vi "录音机实验.vi"() -> ()   [LabVIEW 2011]
uses:
  <vilib>/STM32_DriverVI_Interface_F4/IIC/IIC_Select_F4.ctl
  <vilib>/STM32_DriverVI_Interface_F4/FM/FM Frq Band_F4.ctl
  <vilib>/STM32_DriverVI_Interface_F4/FM/FM Frq Step_F4.ctl
  <vilib>/STM32_DriverVI_Interface_F4/FM/FM RX_TX Mode_F4.ctl
  <vilib>/STM32_DriverVI_Interface_F4/FM/FM Frequency Set_F4.vi
  <vilib>/STM32_DriverVI_Interface_F4/FM/FM Signal Intensity Get_F4.vi
panel:
  out "FM Broadcast Valid?":bool
  in  "自动搜索电台":bool
  out "Signal Intensity（%）":u16
  in  "Volume（%）":u16(slide)=74 max=100 scale=0.0..100.0
  in  "Mute（静音）":bool
  in  "FM Frequency（MHz）":dbl=97.3
  in  "重设电台":bool
  out "Init_Success?":bool
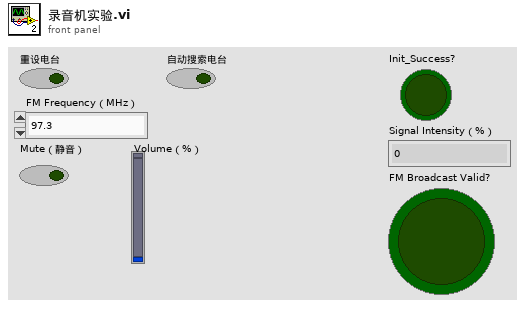
[diagram p1: front panel]
types:
  T1 = typedef "FM RX_TX Mode_F4.ctl" = enum8{"Receive Mode", "Transmit Mode"}
  T2 = typedef "FM Frq Step_F4.ctl" = enum8{"100 KHz", "200 KHz", "50   KHz"}
  T3 = typedef "FM Frq Band_F4.ctl" = enum8{"87MHz~108MHz", "76MHz~91MHz", "76MHz~108MHz"}
  T4 = enum8{"P0", "P1", "P2", "P3", "P4", "P5", "P6", "P7", "P8", "P9", "P10", "P11", "P12", "P13", "P14", "P15"}
  T5 = enum8{"Port_A", "Port_B", "Port_C", "Port_D", "Port_E", "Port_F", "Port_G", "Port_H", "Port_I"}
  T6 = typedef "IIC_Select_F4.ctl" = enum8{"IIC_Group_1", "IIC_Group_2", "IIC_Group_3", "IIC_Group_4", "IIC_Group_5", "IIC_Group_6", "IIC_Group_7", "IIC_Group_8"}
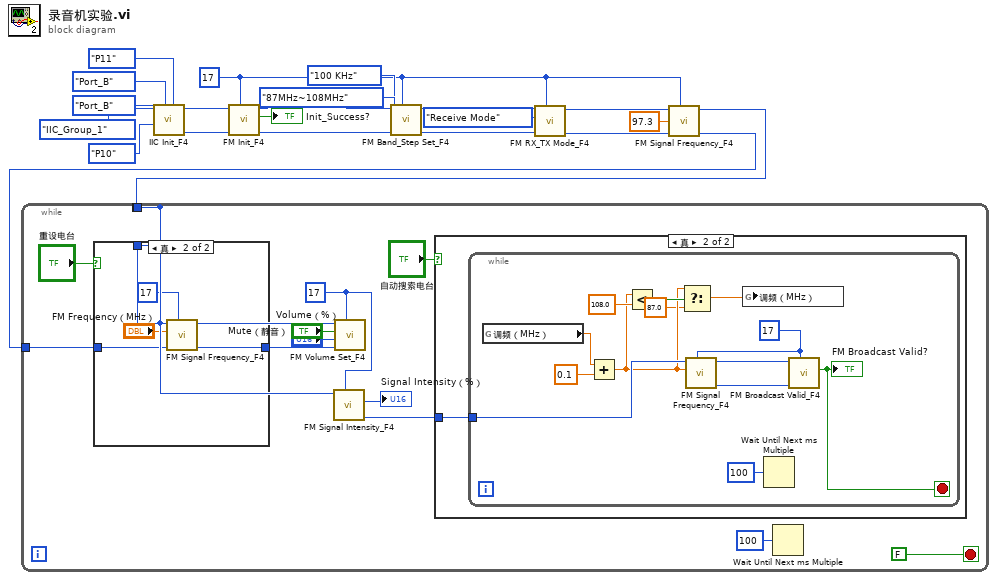
[diagram p0: block diagram]
diagram:
  w3 = u8 17 ("器件地址（7位）")
  n1 = call <vilib>:"IIC Init_F4.vi"("SDA_pin"=T4."P11", "SDA_PortX"=T5."Port_B", "SCL_pin"=T4."P10", "SCL_PortX"=T5."Port_B", "IIC_Select"=IIC_Select_F4."IIC_Group_1") -> ("err_out"=w16:u8, "IIC_Reference_Out"=w15:u16)  [unwired: 5 in]
  n2 = call <vilib>:"FM Init_F4.vi"("器件地址（7位）"=w3, "err_in"=w16, "IIC_Reference_In"=w15) -> ("err_out"=w13:u8, "Init_Success?"=→"Init_Success?":bool, "IIC_Reference_Out"=w12:u16)  [unwired: 6 in]
  n3 = call <vilib>:"FM Band_Step Set_F4.vi"("器件地址（7位）"=w3, "err_in"=w13, "FM Frq Step Set"=FM_Frq_Step_F4."100 KHz", "FM Frq Band Mode"=FM_Frq_Band_F4."87MHz~108MHz", "IIC_Reference_In"=w12) -> ("err_out"=w9:u8, "IIC_Reference_Out"=w8:u16)  [unwired: 5 in]
  n4 = call <vilib>:"FM RX_TX Mode_F4.vi"("器件地址（7位）"=w3, "err_in"=w9, "FM Mode RX/TX"=FM_RX_TX_Mode_F4."Receive Mode", "IIC_Reference_In"=w8) -> ("err_out"=w6:u8, "IIC_Reference_Out"=w5:u16)  [unwired: 6 in]
  n5 = call-poly <vilib>:"FM Signal Frequency_F4.vi"("器件地址（7位）"=w3, "err_in"=w6, "FM Frequency（MHz）"=97.3, "IIC_Reference_In"=w5) -> ("err_out"=w2:u8, "IIC_Reference_Out"=w1:u16)  [unwired: 6 in]
  n6 = while {
    tunnel: w2 -> [w32]
    tunnel: w1 -> [w30]
    tunnel: [w30] -> _
    stop <- FALSE stop-if-true
    w29 = u8 17 ("器件地址（7位）")
    n7 = case shown="真" "重设电台" {
      tunnel: w32 -> [_ w52]
      tunnel: w30 -> [_ w51]
      tunnel: [_ w48] -> w31
      frame False {
      }
      frame True {
        n8 = call-poly <vilib>:"FM Signal Frequency_F4.vi"("器件地址（7位）"=u8 17, "err_in"=w52, "FM Frequency（MHz）"="FM Frequency（MHz）", "IIC_Reference_In"=w51) -> ("err_out"=w48:u8)  [unwired: 6 in, 1 out]
      }
    }
    n9 = call-poly <vilib>:"FM Signal Intensity_F4.vi"("器件地址（7位）"=w29, "IIC_Reference_In"=w30) -> ("err_out"=w22:u8, "Signal Intensity（%）"=→"Signal Intensity（%）":u16)  [unwired: 7 in, 1 out]
    n10 = call <vilib>:"FM Volume Set_F4.vi"("器件地址（7位）"=w29, "err_in"=w31, "Volume（%）"="Volume（%）", "Mute（静音）"="Mute（静音）", "IIC_Reference_In"=w30) -> ()  [unwired: 5 in, 2 out]
    n11 = case shown="真" "自动搜索电台" {
      tunnel: w22 -> [_ w34]
      frame False {
      }
      frame True {
        n12 = while {
          tunnel: w34 -> [w43]
          stop <- w47 stop-if-true
          w44 = u8 17 ("器件地址（7位）")
          n13 = global read "全局变量.vi" "调频（MHz）"() -> (w35:dbl)
          n14 = Add(x=w35, y=0.1) -> (x+y=w38:dbl)
          n15 = Less?(x=w38, y=108.0) -> (x < y?=w39:bool)
          n16 = Select(t=w38, s=w39, f=87.0) -> (s? t:f=w36:dbl)
          n17 = call-poly <vilib>:"FM Signal Frequency_F4.vi"("器件地址（7位）"=w44, "FM Frequency（MHz）"=w38, "IIC_Reference_In"=w43) -> ("err_out"=w46:u8, "IIC_Reference_Out"=w45:u16)  [unwired: 7 in]
          n18 = global write "全局变量.vi" "调频（MHz）"(w36) -> ()
          n19 = Wait Until Next ms Multiple(millisecond multiple=u32 100 ("毫秒倍数")) -> ()  [unwired: 1 out]
          n20 = call <vilib>:"FM Broadcast Valid_F4.vi"("器件地址（7位）"=w44, "err_in"=w46, "IIC_Reference_In"=w45) -> ("FM Broadcast Valid?"=w47:bool)  [unwired: 6 in, 2 out]
          "FM Broadcast Valid?" <- w47
        }
      }
    }
    n21 = Wait Until Next ms Multiple(millisecond multiple=u32 100 ("毫秒倍数")) -> ()  [unwired: 1 out]
  }
